vi "SolenoidTest.vi"() -> ()   [LabVIEW 2013]
uses:
  <vilib>/Rock Robotics/SystemInterfaces/DIO/FPGA_DIOChannel.ctl
  <vilib>/Rock Robotics/SystemInterfaces/Typedef/FPGA_TypedefDigitalModule.ctl
  <vilib>/Rock Robotics/SystemInterfaces/DIO/FPGA_DIORelayChannel.ctl
  <vilib>/Rock Robotics/WPI/Joystick/WPI_JoystickDeviceEnum.ctl
  <vilib>/Rock Robotics/WPI/Solenoid/WPI_SolenoidChannel.ctl
  Robot_Framework_2014/DoubleSolenoidAction.ctl
  Robot_Framework_2014/SingleSolenoidAction.ctl
  <vilib>/Rock Robotics/WPI/Solenoid/WPI_SolenoidOpenSingle.vi
panel:
  in  "Single?":bool
  # "BUTTON 5\nL1"
  # "BUTTON 6\nR1"
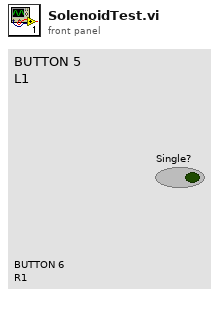
[diagram p1: front panel]
types:
  T1 = typedef "WPI_JoystickDeviceEnum.ctl" = enum16{"USB 1", "USB 2", "USB 3", "USB 4", "Kinect 1", "Kinect 2"}
  T2 = typedef "FPGA_DIORelayChannel.ctl" = enum8{"Relay 1", "Relay 2", "Relay 3", "Relay 4", "Relay 5", "Relay 6", "Relay 7", "Relay 8", "Invalid"}
  T3 = typedef "FPGA_TypedefDigitalModule.ctl" = enum16{"Digital Module 1", "Digital Module 2"}
  T4 = typedef "FPGA_DIOChannel.ctl" = enum8{"DIO 1", "DIO 2", "DIO 3", "DIO 4", "DIO 5", "DIO 6", "DIO 7", "DIO 8", "DIO 9", "DIO 10", "DIO 11", "DIO 12", "DIO 13", "DIO 14", "Invalid"}
  T5 = typedef "WPI_JoystickDevRef.ctl" = cluster{"Device":T1}
  T6 = typedef "DoubleSolenoidAction.ctl" = enum16{"Init", "Middle", "In", "Out"}
  T7 = typedef "WPI_SolenoidChannel.ctl" = enum8{"Solenoid 1", "Solenoid 2", "Solenoid 3", "Solenoid 4", "Solenoid 5", "Solenoid 6", "Solenoid 7", "Solenoid 8", "Invalid"}
  T8 = typedef "SingleSolenoidAction.ctl" = enum16{"Init", "SetState", "Disable"}
  T9 = typedef "WPI_SolenoidDevRef.ctl" = cluster{"DevStatus":errorcluster, "Solenoid Module":T10, "Forward Solenoid Channel":T7, "Reverse Solenoid Channel":T7}
  T10 = typedef "FPGA_TypedefSolenoidModule.ctl" = enum16{"Solenoid Module 1", "Solenoid Module 2"}
  T11 = typedef "WPI_JoystickButtonState.ctl" = cluster{"Button 1":bool, "Button 2":bool, "Button 3":bool, "Button 4":bool, "Button 5":bool, "Button 6":bool, "Button 7":bool, "Button 8":bool, "Button 9":bool, "Button 10":bool, "Button 11":bool, "Button 12":bool}
  T12 = typedef "WPI_CompressorDevRef.ctl" = cluster{"DevStatus":errorcluster, "DigitalInputDevRef":T13, "RelayDevRef":T14}
  T13 = typedef "WPI_DigitalInputDevRef.ctl" = cluster{"DevStatus":errorcluster, "DIO Channel":T4, "Digital Module":T3}
  T14 = typedef "WPI_RelayDevRef.ctl" = cluster{"DevStatus":errorcluster, "Relay Channel":T2, "Digital Module":T3, "Relay Direction":T15}
  T15 = typedef "WPI_RelayDirection.ctl" = enum16{"Both directions", "Forward only", "Reverse only"}
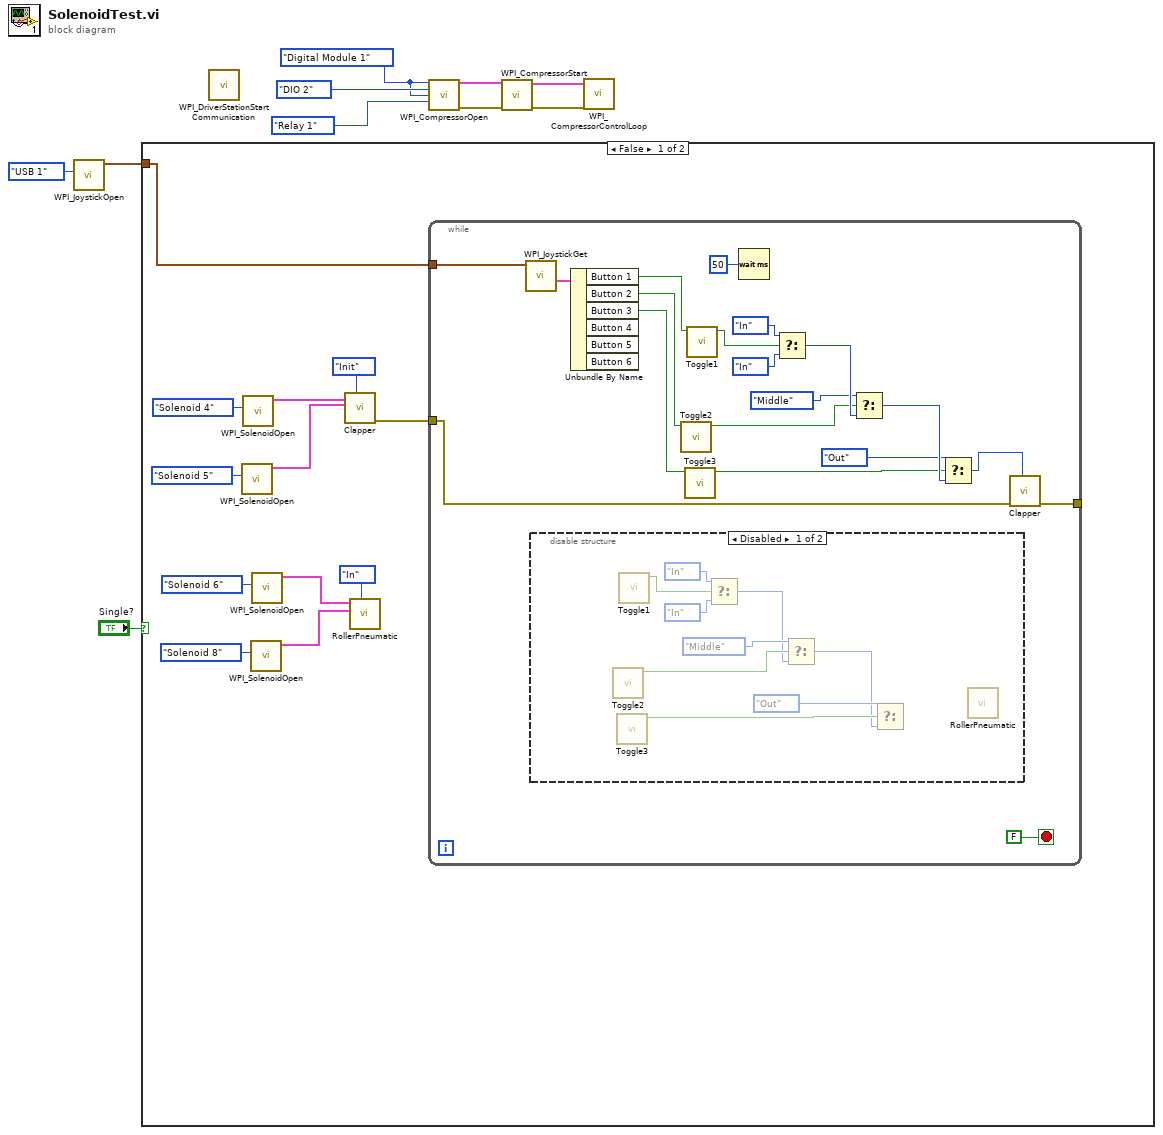
[diagram p0: block diagram]
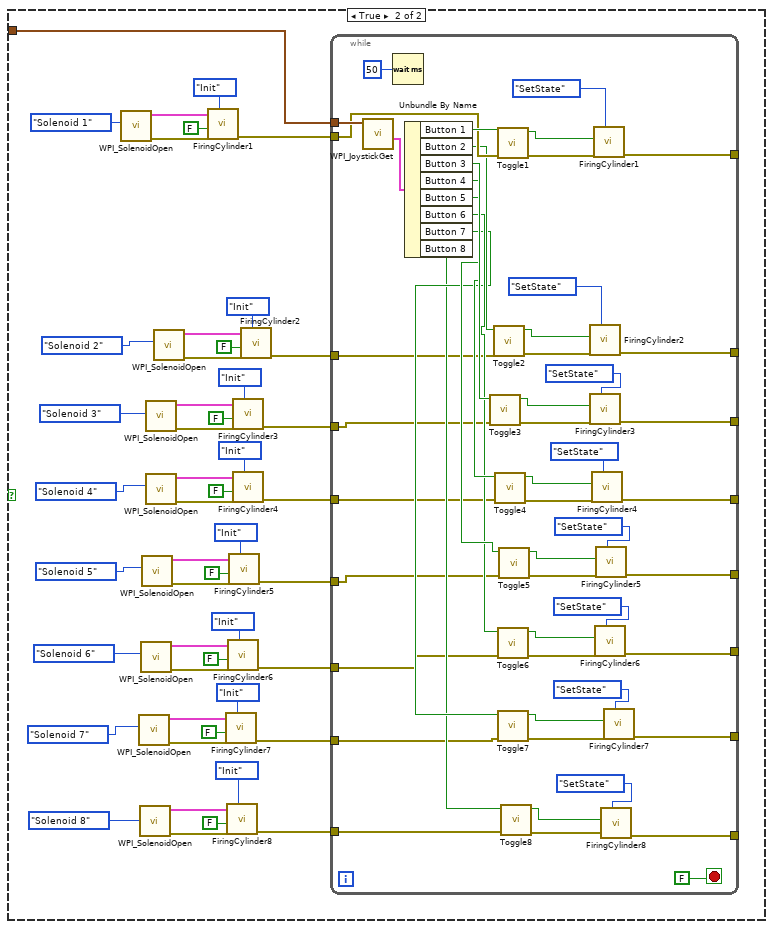
[diagram p3: hidden frame]
diagram:
  w9 = FPGA_TypedefDigitalModule."Digital Module 1" ("Pressure Switch Digital Module (Module 1)")
  n1 = call <vilib>:"WPI_JoystickOpen.vi"("JoystickDevice"=WPI_JoystickDeviceEnum."USB 1") -> ("JoystickDevRef"=w1:T5)  [unwired: 10 in]
  n2 = case shown="False" "Single?" {
    tunnel: w1 -> [w17 w54]
    frame False {
      n3 = call-poly <vilib>:"WPI_SolenoidOpen.vi"("Solenoid Channel"=WPI_SolenoidChannel."Solenoid 5") -> ("SolenoidDevRef"=w19:T9)  [unwired: 9 in, 1 out]
      n4 = call-poly <vilib>:"WPI_SolenoidOpen.vi"("Solenoid Channel"=WPI_SolenoidChannel."Solenoid 4") -> ("SolenoidDevRef"=w20:T9)  [unwired: 9 in, 1 out]
      n5 = call-poly <vilib>:"WPI_SolenoidOpen.vi"("Solenoid Channel"=WPI_SolenoidChannel."Solenoid 8") -> ("SolenoidDevRef"=w13:T9)  [unwired: 9 in, 1 out]
      n6 = call-poly <vilib>:"WPI_SolenoidOpen.vi"("Solenoid Channel"=WPI_SolenoidChannel."Solenoid 6") -> ("SolenoidDevRef"=w12:T9)  [unwired: 9 in, 1 out]
      n7 = call "Clapper.vi"("State"=DoubleSolenoidAction."Init", "Plugged"=w19, "Open"=w20) -> ("Error out"=w18:errorcluster)  [unwired: 8 in]
      n8 = call "RollerPneumatic.vi"("State"=DoubleSolenoidAction."In", "Plugged"=w13, "Open"=w12) -> ()  [unwired: 8 in, 1 out]
      n9 = while {
        tunnel: w18 -> [w24]
        tunnel: w17 -> [w39]
        tunnel: [w23] -> _
        stop <- FALSE stop-if-true
        n10 = call <vilib>:"WPI_JoystickGet.vi"("JoystickDevRef"=w39) -> ("Buttons"=w37:T11)  [unwired: 4 in, 2 out]
        n11 = disable-structure shown="Disabled" {
          frame Disabled {
            n12 = call "Toggle2.vi"() -> ("ToggleState"=w50:bool, "RawInput"=w44:bool)  [unwired: 9 in, 1 out]
            n13 = call "Toggle3.vi"() -> ("ToggleState"=w53:bool, "RawInput"=w45:bool)  [unwired: 9 in, 1 out]
            n14 = call "Toggle1.vi"() -> ("ToggleState"=w42:bool, "RawInput"=w43:bool)  [unwired: 9 in, 1 out]
            n15 = Select(t=DoubleSolenoidAction."In" ("State"), s=w42, f=DoubleSolenoidAction."In" ("State")) -> (s? t:f=w48:T6)
            n16 = Select(t=DoubleSolenoidAction."Middle" ("State"), s=w50, f=w48) -> (s? t:f=w51:T6)
            n17 = Select(t=DoubleSolenoidAction."Out" ("State"), s=w53, f=w51) -> ()  [unwired: 1 out]
            n18 = call "RollerPneumatic.vi"() -> ()  [unwired: 11 in, 1 out]
          }
          frame Enabled {
          }
        }
        n19 = Unbundle By Name(w37) -> ("Button 1"=w36:bool, "Button 2"=w35:bool, "Button 3"=w34:bool)  [unwired: 3 out]
        n20 = call "Toggle2.vi"("RawInput"=w35) -> ("ToggleState"=w29:bool)  [unwired: 9 in, 1 out]
        n21 = call "Toggle3.vi"("RawInput"=w34) -> ("ToggleState"=w26:bool)  [unwired: 9 in, 1 out]
        n22 = call "Toggle1.vi"("RawInput"=w36) -> ("ToggleState"=w38:bool)  [unwired: 9 in, 1 out]
        n23 = Wait (ms)(milliseconds to wait=u32 50) -> ()  [unwired: 1 out]
        n24 = Select(t=DoubleSolenoidAction."In" ("State"), s=w38, f=DoubleSolenoidAction."In" ("State")) -> (s? t:f=w31:T6)
        n25 = Select(t=DoubleSolenoidAction."Middle" ("State"), s=w29, f=w31) -> (s? t:f=w28:T6)
        n26 = Select(t=DoubleSolenoidAction."Out" ("State"), s=w26, f=w28) -> (s? t:f=w25:T6)
        n27 = call "Clapper.vi"("State"=w25, "Error in"=w24) -> ("Error out"=w23:errorcluster)  [unwired: 9 in]
      }
    }
    frame True {
      n28 = call-poly <vilib>:"WPI_SolenoidOpen.vi"("Solenoid Channel"=WPI_SolenoidChannel."Solenoid 1") -> ("error out"=w98:errorcluster, "SolenoidDevRef"=w99:T9)  [unwired: 9 in]
      n29 = call-poly <vilib>:"WPI_SolenoidOpen.vi"("Solenoid Channel"=WPI_SolenoidChannel."Solenoid 7") -> ("error out"=w78:errorcluster, "SolenoidDevRef"=w77:T9)  [unwired: 9 in]
      n30 = call-poly <vilib>:"WPI_SolenoidOpen.vi"("Solenoid Channel"=WPI_SolenoidChannel."Solenoid 8") -> ("error out"=w73:errorcluster, "SolenoidDevRef"=w74:T9)  [unwired: 9 in]
      n31 = call-poly <vilib>:"WPI_SolenoidOpen.vi"("Solenoid Channel"=WPI_SolenoidChannel."Solenoid 6") -> ("error out"=w79:errorcluster, "SolenoidDevRef"=w80:T9)  [unwired: 9 in]
      n32 = call-poly <vilib>:"WPI_SolenoidOpen.vi"("Solenoid Channel"=WPI_SolenoidChannel."Solenoid 5") -> ("error out"=w85:errorcluster, "SolenoidDevRef"=w84:T9)  [unwired: 9 in]
      n33 = call-poly <vilib>:"WPI_SolenoidOpen.vi"("Solenoid Channel"=WPI_SolenoidChannel."Solenoid 3") -> ("error out"=w93:errorcluster, "SolenoidDevRef"=w92:T9)  [unwired: 9 in]
      n34 = call-poly <vilib>:"WPI_SolenoidOpen.vi"("Solenoid Channel"=WPI_SolenoidChannel."Solenoid 4") -> ("error out"=w86:errorcluster, "SolenoidDevRef"=w87:T9)  [unwired: 9 in]
      n35 = call-poly <vilib>:"WPI_SolenoidOpen.vi"("Solenoid Channel"=WPI_SolenoidChannel."Solenoid 2") -> ("error out"=w94:errorcluster, "SolenoidDevRef"=w95:T9)  [unwired: 9 in]
      n36 = call "FiringCylinder1.vi"("Action"=SingleSolenoidAction."Init", "error in (no error)"=w98, "Default Position"=FALSE, "SolenoidDevRef"=w99) -> ("error out"=w101:errorcluster)  [unwired: 7 in]
      n37 = call "FiringCylinder7.vi"("Action"=SingleSolenoidAction."Init", "error in (no error)"=w78, "Default Position"=FALSE, "SolenoidDevRef"=w77) -> ("error out"=w67:errorcluster)  [unwired: 7 in]
      n38 = call "FiringCylinder8.vi"("Action"=SingleSolenoidAction."Init", "error in (no error)"=w73, "Default Position"=FALSE, "SolenoidDevRef"=w74) -> ("error out"=w66:errorcluster)  [unwired: 7 in]
      n39 = call "FiringCylinder6.vi"("Action"=SingleSolenoidAction."Init", "error in (no error)"=w79, "Default Position"=FALSE, "SolenoidDevRef"=w80) -> ("error out"=w68:errorcluster)  [unwired: 7 in]
      n40 = call "FiringCylinder5.vi"("Action"=SingleSolenoidAction."Init", "error in (no error)"=w85, "Default Position"=FALSE, "SolenoidDevRef"=w84) -> ("error out"=w69:errorcluster)  [unwired: 7 in]
      n41 = call "FiringCylinder3.vi"("Action"=SingleSolenoidAction."Init", "error in (no error)"=w93, "Default Position"=FALSE, "SolenoidDevRef"=w92) -> ("error out"=w71:errorcluster)  [unwired: 7 in]
      n42 = call "FiringCylinder4.vi"("Action"=SingleSolenoidAction."Init", "error in (no error)"=w86, "Default Position"=FALSE, "SolenoidDevRef"=w87) -> ("error out"=w70:errorcluster)  [unwired: 7 in]
      n43 = call "FiringCylinder2.vi"("Action"=SingleSolenoidAction."Init", "error in (no error)"=w94, "Default Position"=FALSE, "SolenoidDevRef"=w95) -> ("error out"=w72:errorcluster)  [unwired: 7 in]
      n44 = while {
        tunnel: w101 -> [w149]
        tunnel: w54 -> [w153]
        tunnel: w72 -> [w135]
        tunnel: w71 -> [w136]
        tunnel: w70 -> [w137]
        tunnel: w69 -> [w138]
        tunnel: w68 -> [w139]
        tunnel: w67 -> [w140]
        tunnel: w66 -> [w141]
        tunnel: [w132] -> _
        tunnel: [w127] -> _
        tunnel: [w125] -> _
        tunnel: [w120] -> _
        tunnel: [w116] -> _
        tunnel: [w112] -> _
        tunnel: [w108] -> _
        tunnel: [w104] -> _
        stop <- FALSE stop-if-true
        n45 = call <vilib>:"WPI_JoystickGet.vi"("JoystickDevRef"=w153) -> ("Buttons"=w152:T11)  [unwired: 4 in, 2 out]
        n46 = Wait (ms)(milliseconds to wait=u32 50) -> ()  [unwired: 1 out]
        n47 = Unbundle By Name(w152) -> ("Button 1"=w151:bool, "Button 2"=w148:bool, "Button 3"=w147:bool, "Button 4"=w146:bool, "Button 5"=w145:bool, "Button 6"=w144:bool, "Button 7"=w143:bool, "Button 8"=w142:bool)
        n48 = call "Toggle3.vi"("error in"=w136, "RawInput"=w147) -> ("error out"=w126:errorcluster, "ToggleState"=w123:bool)  [unwired: 8 in]
        n49 = call "Toggle2.vi"("error in"=w135, "RawInput"=w148) -> ("error out"=w128:errorcluster, "ToggleState"=w129:bool)  [unwired: 8 in]
        n50 = call "Toggle4.vi"("error in"=w137, "RawInput"=w146) -> ("error out"=w121:errorcluster, "ToggleState"=w119:bool)  [unwired: 8 in]
        n51 = call "Toggle1.vi"("error in"=w149, "RawInput"=w151) -> ("error out"=w134:errorcluster, "ToggleState"=w133:bool)  [unwired: 8 in]
        n52 = call "Toggle6.vi"("error in"=w139, "RawInput"=w144) -> ("error out"=w113:errorcluster, "ToggleState"=w111:bool)  [unwired: 8 in]
        n53 = call "Toggle7.vi"("error in"=w140, "RawInput"=w143) -> ("error out"=w109:errorcluster, "ToggleState"=w107:bool)  [unwired: 8 in]
        n54 = call "Toggle5.vi"("error in"=w138, "RawInput"=w145) -> ("error out"=w117:errorcluster, "ToggleState"=w115:bool)  [unwired: 8 in]
        n55 = call "Toggle8.vi"("error in"=w141, "RawInput"=w142) -> ("error out"=w105:errorcluster, "ToggleState"=w103:bool)  [unwired: 8 in]
        n56 = call "FiringCylinder2.vi"("Action"=SingleSolenoidAction."SetState", "error in (no error)"=w128, "Actuate?"=w129) -> ("error out"=w127:errorcluster)  [unwired: 8 in]
        n57 = call "FiringCylinder3.vi"("Action"=SingleSolenoidAction."SetState", "error in (no error)"=w126, "Actuate?"=w123) -> ("error out"=w125:errorcluster)  [unwired: 8 in]
        n58 = call "FiringCylinder4.vi"("Action"=SingleSolenoidAction."SetState", "error in (no error)"=w121, "Actuate?"=w119) -> ("error out"=w120:errorcluster)  [unwired: 8 in]
        n59 = call "FiringCylinder1.vi"("Action"=SingleSolenoidAction."SetState", "error in (no error)"=w134, "Actuate?"=w133) -> ("error out"=w132:errorcluster)  [unwired: 8 in]
        n60 = call "FiringCylinder6.vi"("Action"=SingleSolenoidAction."SetState", "error in (no error)"=w113, "Actuate?"=w111) -> ("error out"=w112:errorcluster)  [unwired: 8 in]
        n61 = call "FiringCylinder5.vi"("Action"=SingleSolenoidAction."SetState", "error in (no error)"=w117, "Actuate?"=w115) -> ("error out"=w116:errorcluster)  [unwired: 8 in]
        n62 = call "FiringCylinder8.vi"("Action"=SingleSolenoidAction."SetState", "error in (no error)"=w105, "Actuate?"=w103) -> ("error out"=w104:errorcluster)  [unwired: 8 in]
        n63 = call "FiringCylinder7.vi"("Action"=SingleSolenoidAction."SetState", "error in (no error)"=w109, "Actuate?"=w107) -> ("error out"=w108:errorcluster)  [unwired: 8 in]
      }
    }
  }
  n64 = call <vilib>:"WPI_DriverStationStart Communication.vi"() -> ()  [unwired: 12 in]
  n65 = call <vilib>:"WPI_CompressorOpen.vi"("Pressure Switch Digital Module (Module 1)"=w9, "Pressure Switch DIO Channel"=FPGA_DIOChannel."DIO 2", "Relay Digital Module (Module 1)"=w9, "Relay Channel"=FPGA_DIORelayChannel."Relay 1") -> ("CompressorDevRef"=w7:T12, "error out"=w6:errorcluster)  [unwired: 10 in]
  n66 = call <vilib>:"WPI_CompressorStart.vi"("error in (no error)"=w6, "CompressorDevRef"=w7) -> ("error out"=w5:errorcluster, "CompressorDevRef"=w4:T12)  [unwired: 8 in]
  n67 = call <vilib>:"WPI_CompressorControlLoop.vi"("error in (no error)"=w5, "CompressorDevRef"=w4) -> ()  [unwired: 10 in]
